vi "Update Name.vi"(8 "error in (no error)":errorcluster, 10 "Time Stamp":timestamp, 11 "File in":refnum<class "File.lvclass">) -> (0 "error out":errorcluster, 3 "File out":refnum<class "File.lvclass">)   [LabVIEW 2024, in "File.lvclass"]
uses:
  File.lvclass
  File.lvclass/File.ctl
  Write Data File  Path.vi
  Write Settings File Path.vi
  Write Index  File Path.vi
  Write Index.vi
  Read Include time.vi
  Read File format.vi
  Read Root Data Folder.vi
  Read Project folder .vi
  Read Index digits.vi
  Read File Prefix.vi
  Read File middle.vi
  Read Data File  Path.vi
  Read Settings File Path.vi
  Read Index  File Path.vi
  Read Index.vi
  Read Index file.vi
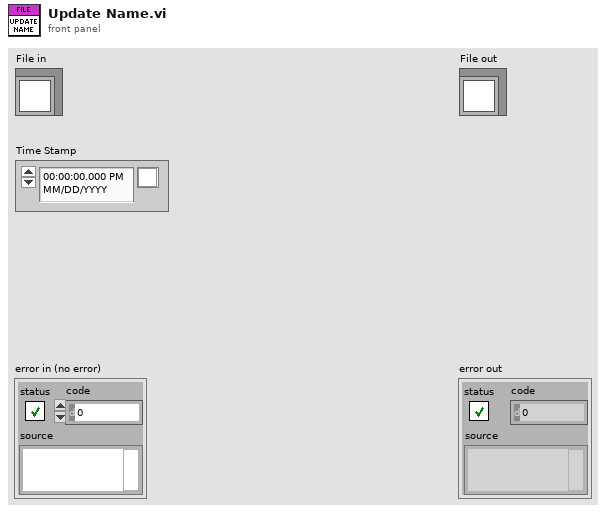
[diagram p1: front panel]
types:
  T1 = typedef "File formats.ctl" = enum16{"TDMS", "ASCII", "BINARY"}
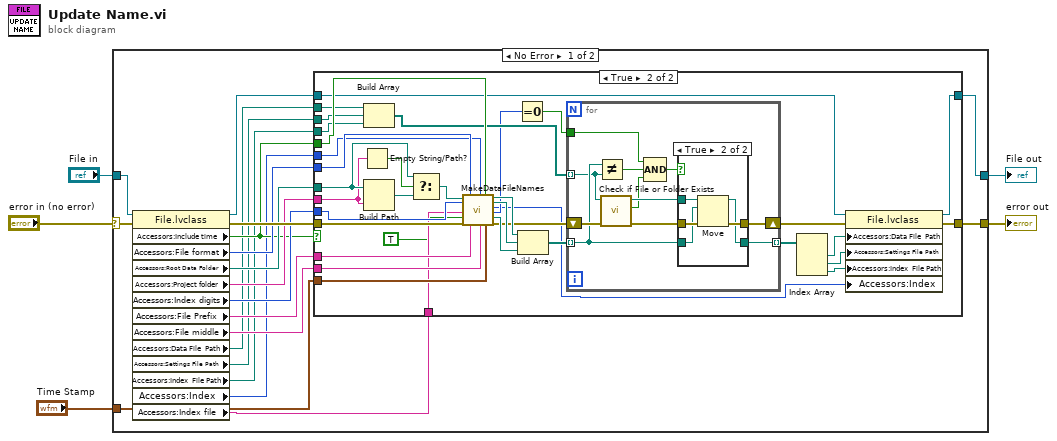
[diagram p0: block diagram]
diagram:
  n1 = case shown="No Error" "error in (no error)" {
    selector: "error in (no error)" -> [w16 w81]
    tunnel: [w9 w81] -> w4
    tunnel: [w10 w80] -> w2
    tunnel: "File in" -> [w17 w80]
    tunnel: "Time Stamp" -> [w8 _]
    frame No Error {
      n2 = property class="File.lvclass"(reference=w17, error in=w16) -> (reference out=w11:refnum<class "File.lvclass">, error out=w24:errorcluster, "Accessors:Include time"=w15:bool, "Accessors:File format"=w22:T1, "Accessors:Root Data Folder"=w20:path, "Accessors:Project folder "=w19:string, "Accessors:Index digits"=w21:i32, "Accessors:File Prefix"=w23:string, "Accessors:File middle"=w18:string, "Accessors:Data File  Path"=w14:path, "Accessors:Settings File Path"=w13:path, "Accessors:Index  File Path"=w12:path, "Accessors:Index"=w7:i32, "Accessors:Index file"=w6:string)
      n3 = case shown="True" w15 {
        tunnel: w24 -> [w25 w61]
        tunnel: w23 -> [_ w60]
        tunnel: w15 -> [_ w59]
        tunnel: w22 -> [_ w58]
        tunnel: w21 -> [_ w57]
        tunnel: w20 -> [_ w55]
        tunnel: w19 -> [_ w54]
        tunnel: w18 -> [_ w51]
        tunnel: w14 -> [_ w50]
        tunnel: w13 -> [_ w49]
        tunnel: w12 -> [_ w48]
        tunnel: w11 -> [w26 w40]
        tunnel: [w26 w35] -> w10
        tunnel: [w25 w34] -> w9
        tunnel: w8 -> [_ w33]
        tunnel: w7 -> [_ w30]
        tunnel: w6 -> [_ w29]
        frame False {
        }
        frame True {
          n4 = Empty String/Path?(string/path=w54) -> (empty?=w56:bool)
          n5 = Build Array(w50, w49, w48) -> (w43:path[])
          n6 = Build Path(base path=w55, name or relative path=w54) -> (appended path=w53:path)
          n7 = Select(t=w55, s=w56, f=w53) -> (s? t:f=w52:path)
          n8 = call "MakeDataFileNames.vi"("Root Data Folder"=w52, "Index digits"=w57, "Index file"=w29, "Interactive"=TRUE, "Error In"=w61, "File format"=w58, "File Prefix"=w60, "Re-use index"=w30, "File middle"=w51, "Include time"=w59, "Time Stamp (default 0 = now)"=w33) -> ("Data File  Path"=w47:path, "Settings File Path"=w46:path, "Index out"=w27:i32, "Try count"=w32:i32, "Index  File Path"=w45:path, "Error Out"=w42:errorcluster)  [unwired: 3 in]
          n9 = Equal To 0?(x=w32) -> (x = 0?=w31:bool)
          n10 = Build Array(w47, w46, w45) -> (w44:path[])
          n11 = for {
            tunnel: w44 -> [w67] mode=indexing
            tunnel: w43 -> [w66] mode=indexing
            shift-right: [w69] -> w36
            shift-left: w42 -> [w72]
            tunnel: [w68] -> w41 mode=indexing
            tunnel: w31 -> [w62]
            n12 = Not Equal?(x=w67, y=w66) -> (x != y?=w63:bool)
            n13 = call <vilib>:"Check if File or Folder Exists.vi"("error in (no error)"=w72, "path"=w66) -> ("error out"=w71:errorcluster, "file or folder exists?"=w64:bool, "dup path"=w70:path)  [unwired: 7 in]
            n14 = Compound Arithmetic op=AND(w62, w63, w64) -> (w65:bool)
            n15 = case shown="True" w65 {
              tunnel: w71 -> [w73 w79]
              tunnel: w70 -> [_ w78]
              tunnel: w67 -> [w74 w77]
              tunnel: [w73 w76] -> w69
              tunnel: [w74 w75] -> w68
              frame False {
              }
              frame True {
                n16 = Move(source path=w78, error in=w79, 10:w77) -> (error out=w76:errorcluster, 3:w75:path)  [unwired: 2 in, 1 out]
              }
            }
          }
          n17 = Index Array(array=w41) -> (element #1=w39:path, element #2=w38:path, element #3=w37:path)  [unwired: 3 in]
          n18 = property class="File.lvclass"(reference=w40, error in=w36, "Accessors:Data File  Path"=w39, "Accessors:Settings File Path"=w38, "Accessors:Index  File Path"=w37, "Accessors:Index"=w27) -> (reference out=w35:refnum<class "File.lvclass">, error out=w34:errorcluster)
        }
      }
    }
    frame Error {
    }
  }
  "error out" <- w4
  "File out" <- w2
